vi "UICtrls_Write_Name_(poly).vi"   [LabVIEW 2025]
uses:
  UI_Manager/UI_Manager.lvclass
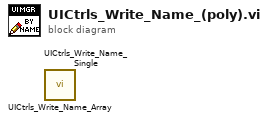
[diagram p0: block diagram]
diagram:
  n1 = call "UICtrls_Write_Name_Array.vi"() -> ()  [unwired: 10 in, 2 out]
  n2 = call "UICtrls_Write_Name_Single.vi"() -> ()  [unwired: 10 in, 2 out]
